vi "Main.vi"() -> ()   [LabVIEW 2018, in "Application.lvlib"]
doc: "This VI is the main application VI in the Delacor QMH project template. This application VI is implemented as a simple state machine, which communicates with two different Delacor QMH modules.\n_____\nBased on DQMH Project Template 6.0.0.91."
uses:
  Application.lvlib
  Application Data--cluster.ctl
  State--enum.ctl
  CE14 eMIC module/CE14 eMIC module.lvlib
  Switches Module/Switches Module.lvlib
panel:
  in  "Array":bool[](array[boolean])
  in  "MB01":bool
  in  "CloseCOM":bool
  in  "OpenCOM":bool
  out "version":string
  in  "Hide Switches Module Module":bool
  in  "Show Switches Module Module":bool
  in  "Hide CE14 eMIC module Module":bool
  in  "Show CE14 eMIC module Module":bool
  in  "Stop CE14 eMIC module Module":bool
  in  "Stop Switches Module Module":bool
  in  "Start Switches Module Module":bool
  out "Active CE14 eMIC module Modules":string[](array[string])
  in  "Start New Instance CE14 eMIC module Module":bool
  in  "Select CE14 eMIC module Module Instance":i32(ring)=-1 items=["All"=-1]
  in  "Switches Module Module: Do Something Else":dbl caption="Do Something Else"
  in  "Switches Module Module: Do Something":bool
  out "Switches Module Running?":bool
  out "Status":string
  in  "CE14 eMIC module Module: Do Something Else":dbl caption="Do Something Else to Selected Module"
  in  "CE14 eMIC module Module: Do Something":bool caption="Do Something to Selected Module"
  # "This top-level application allows you to launch and control a singleton module, and multiple instances of a cloneable module."
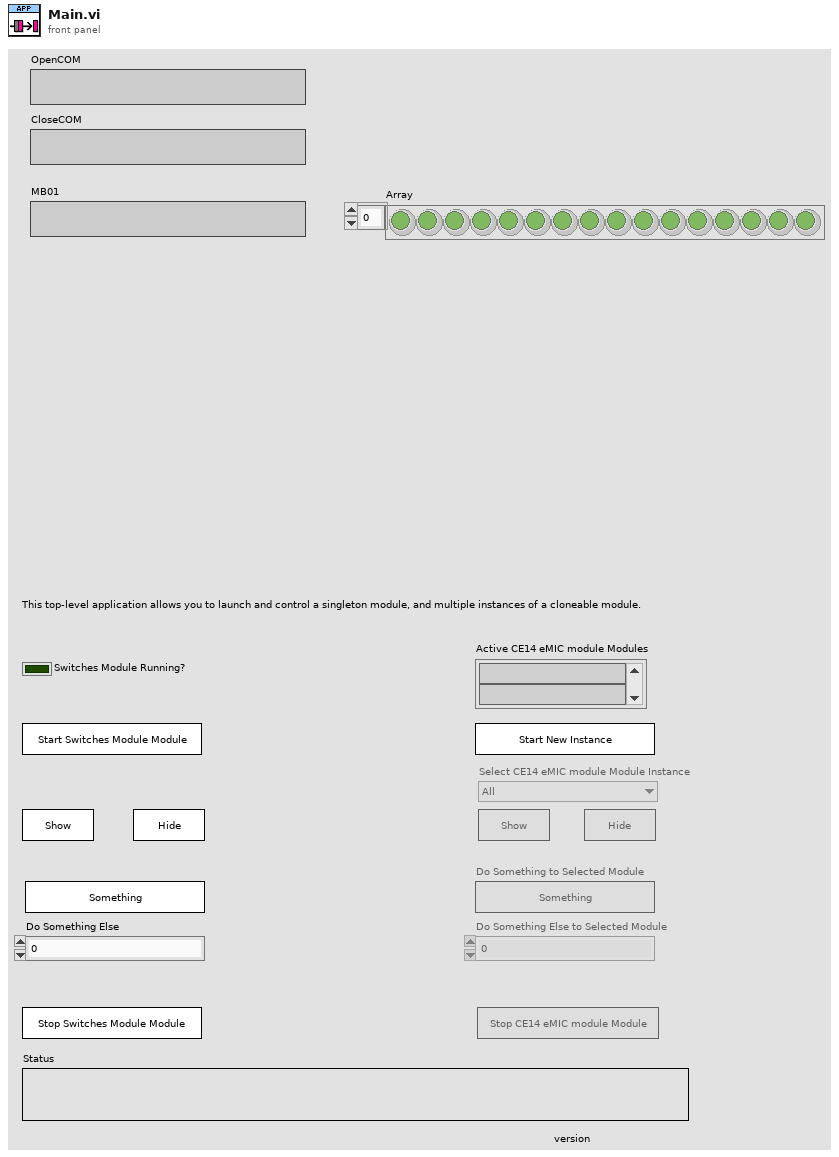
[diagram p1: front panel]
types:
  T1 = typedef "Application.lvlib/State--enum.ctl" = enum16{"Initialize", "Initialize Panel", "UI Interlocks", "Update Status", "Wait for Event", "Exit"}
  T2 = typedef "Application.lvlib/Application Data--cluster.ctl" = cluster{"Status":string, "Singleton Controls":refnum<vi>[], "Cloneable Controls":refnum<vi>[], "Module Ring Value":i32}
  T3 = typedef "CE14 eMIC module.lvlib/Broadcast Events--cluster.ctl" = cluster{"Module Did Init":refnum<user-event>, "Status Updated":refnum<user-event>, "Error Reported":refnum<user-event>, "Did Something":refnum<user-event>, "Module Did Stop":refnum<user-event>, "Update Module Execution Status":refnum<user-event>}
  T4 = typedef "Switches Module.lvlib/Broadcast Events--cluster.ctl" = cluster{"Module Did Init":refnum<user-event>, "Status Updated":refnum<user-event>, "Error Reported":refnum<user-event>, "Did Something":refnum<user-event>, "Module Did Stop":refnum<user-event>, "Update Module Execution Status":refnum<user-event>}
  T5 = enum8{"Enabled", "Disabled", "Disabled and Grayed Out"}
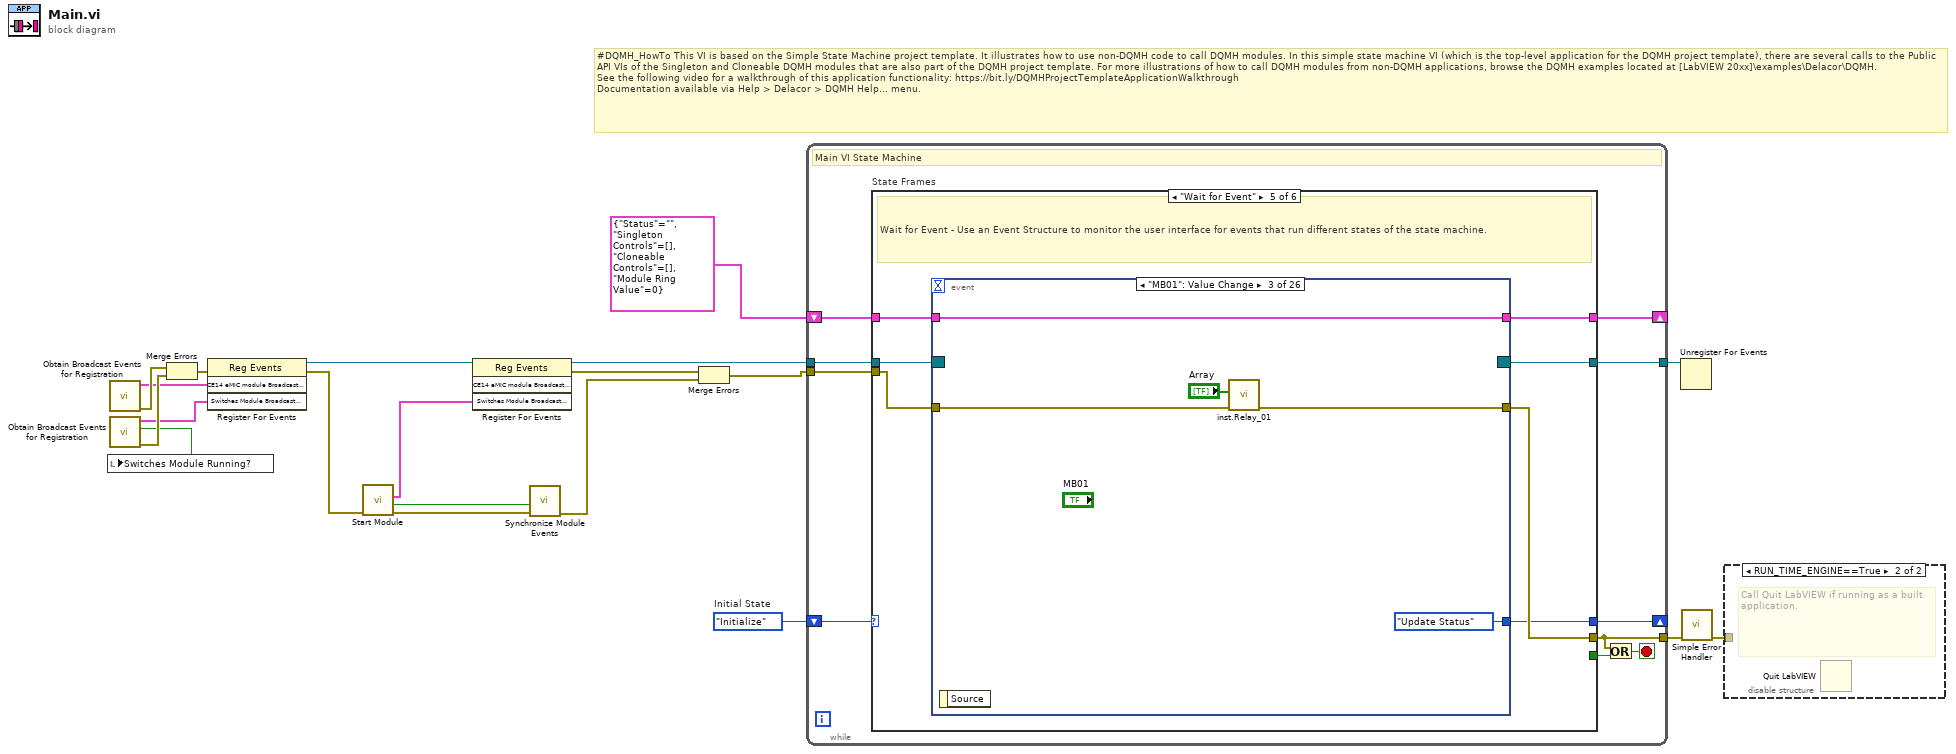
[diagram p0: block diagram]
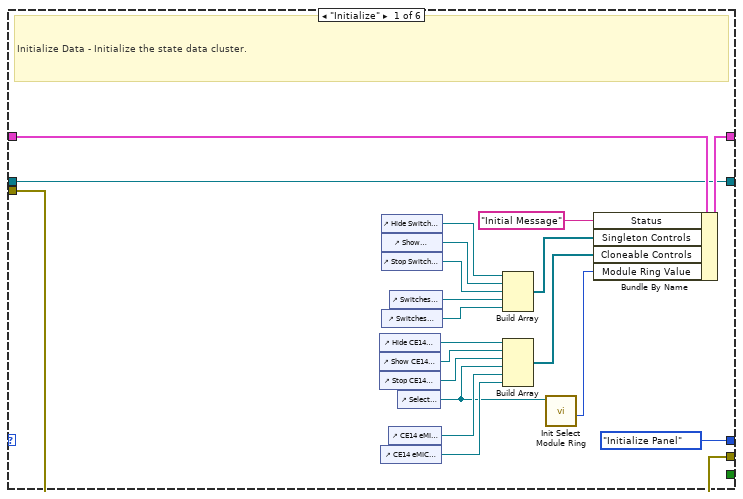
[diagram p2: hidden frame]
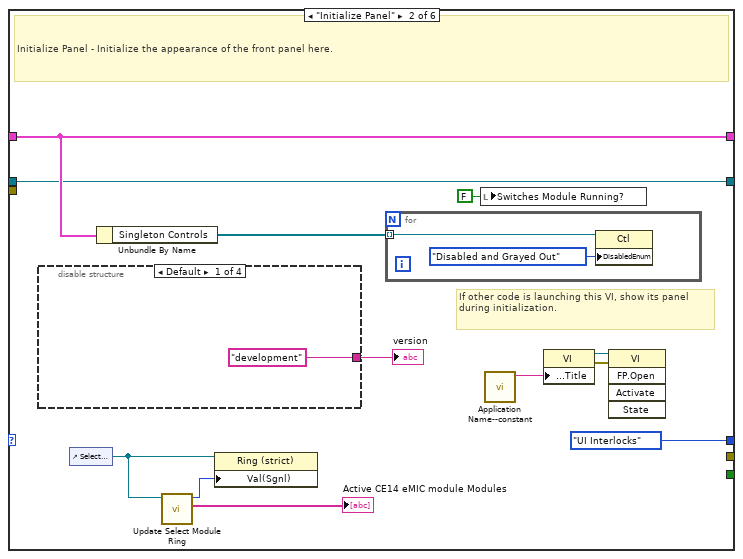
[diagram p3: hidden frame]
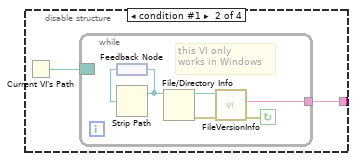
[diagram p4: hidden frame]
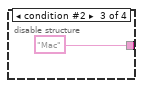
[diagram p5: hidden frame]
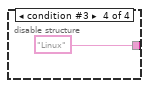
[diagram p6: hidden frame]
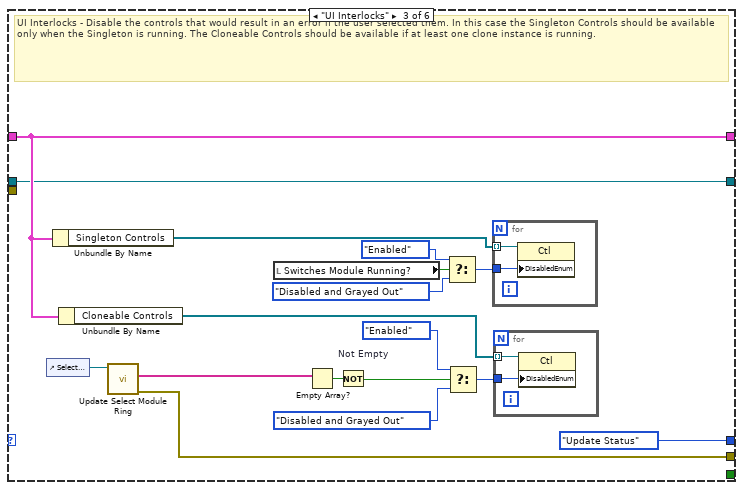
[diagram p7: hidden frame]
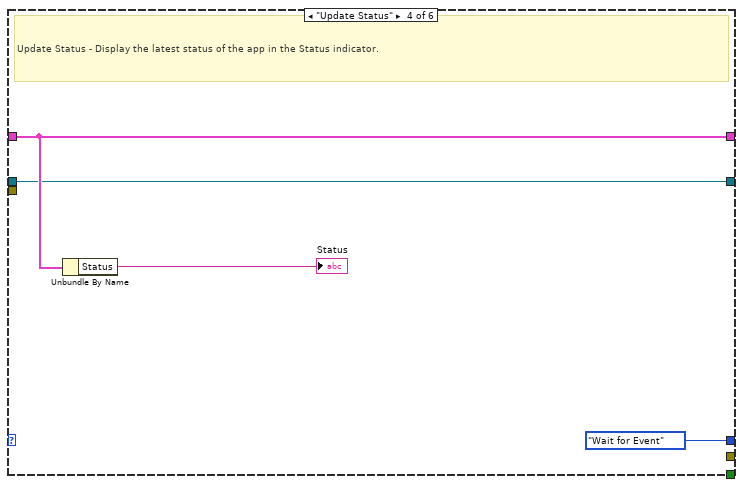
[diagram p8: hidden frame]
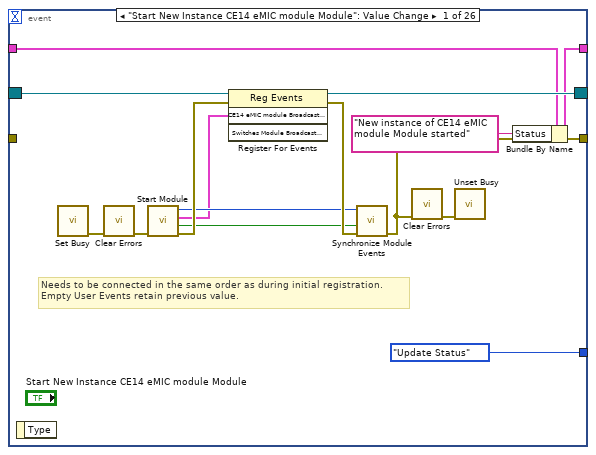
[diagram p9: hidden frame]
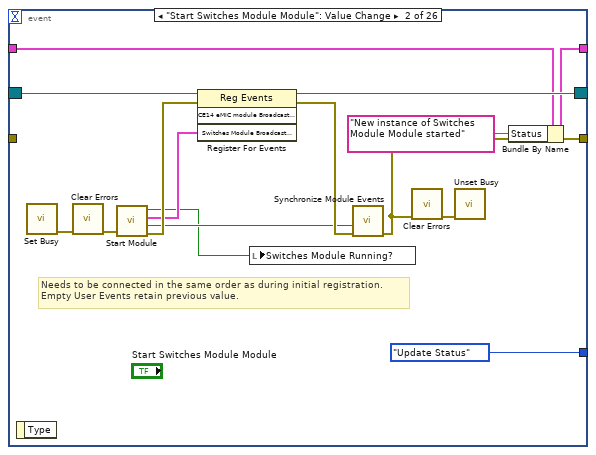
[diagram p10: hidden frame]
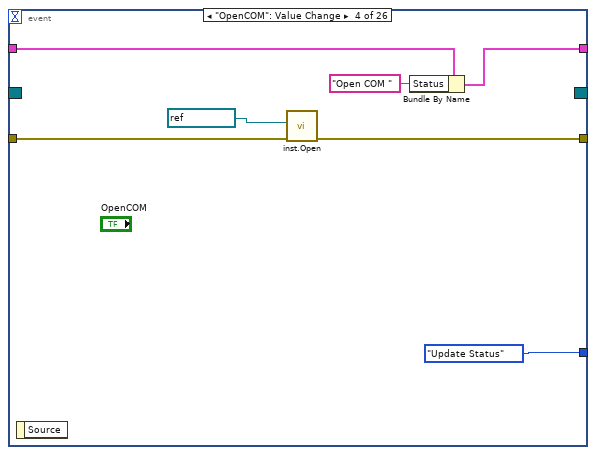
[diagram p11: hidden frame]
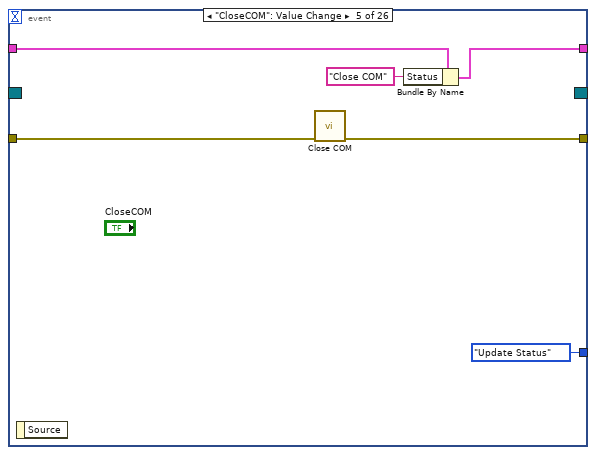
[diagram p12: hidden frame]
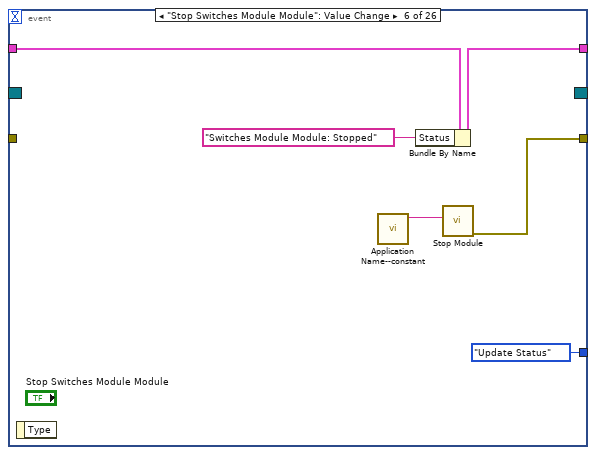
[diagram p13: hidden frame]
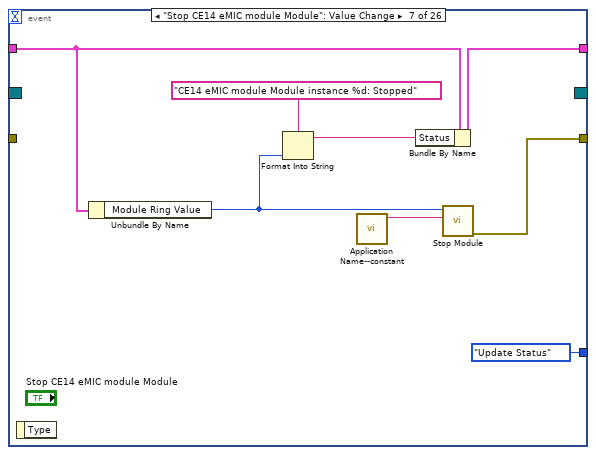
[diagram p14: hidden frame]
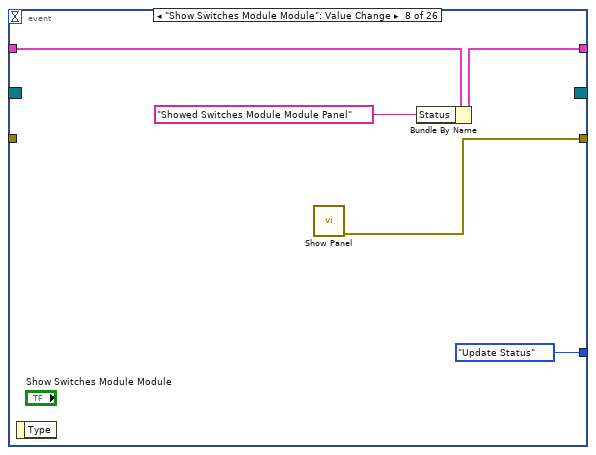
[diagram p15: hidden frame]
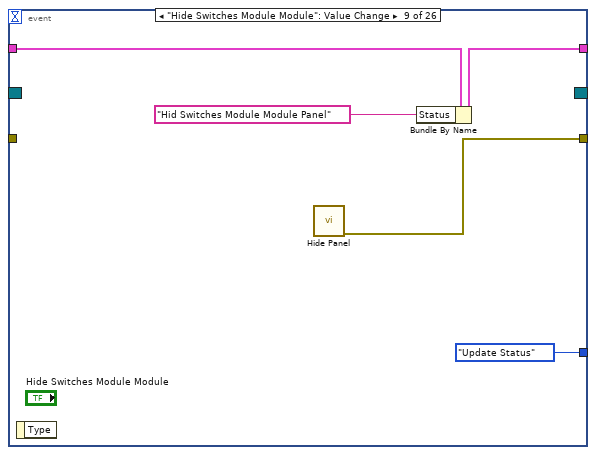
[diagram p16: hidden frame]
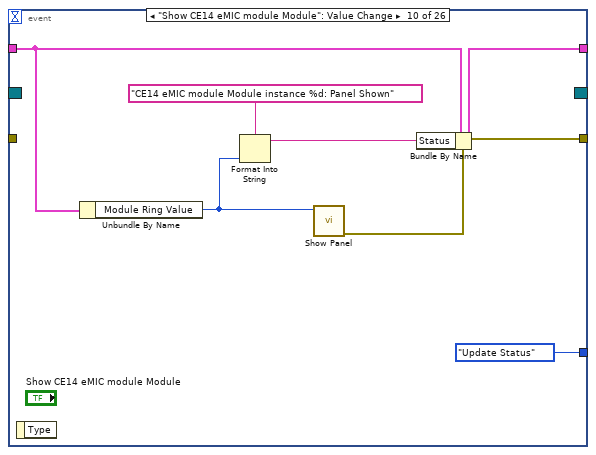
[diagram p17: hidden frame]
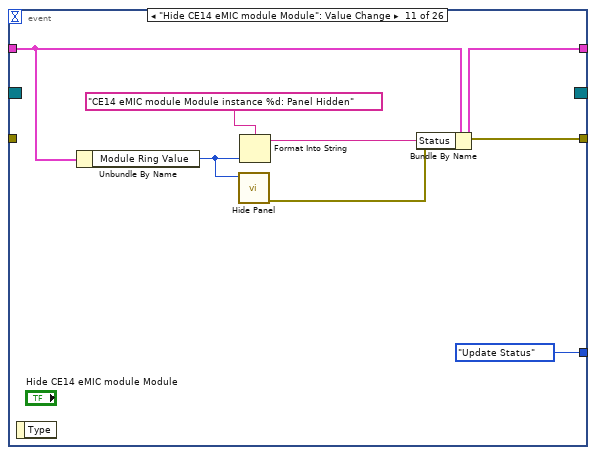
[diagram p18: hidden frame]
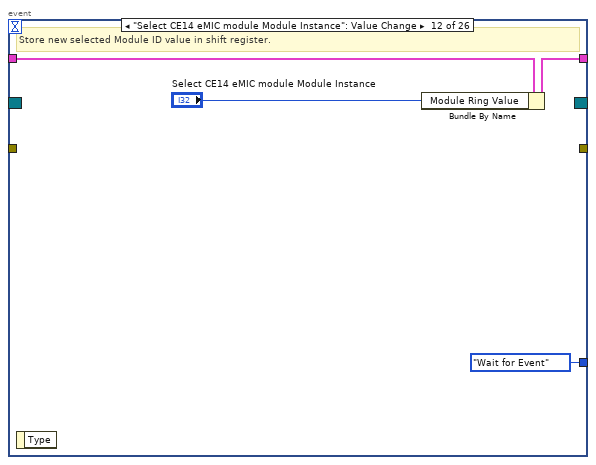
[diagram p19: hidden frame]
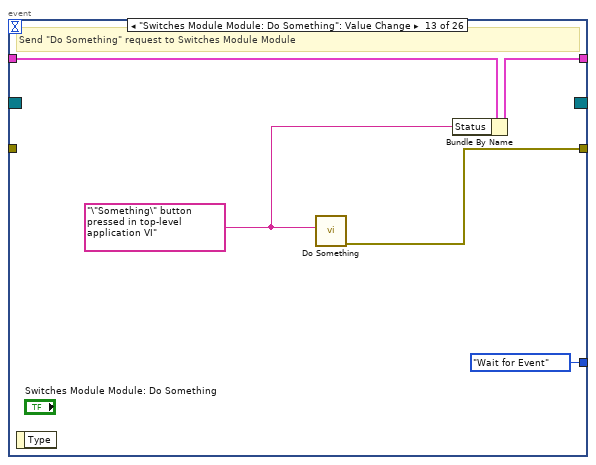
[diagram p20: hidden frame]
diagram:
  w12 = State--enum."Initialize"  # Initial State
  # "#DQMH_HowTo This VI is based on the Simple State Machine project template. It illustrates how to use non-DQMH code to call DQMH modules. In this simple state machine VI (which is the top-level application for the DQMH project template), there are several calls to the Public API VIs of the Singleton and Cloneable DQMH modules that are also part of the DQMH project template. For more illustrations of how to call DQMH modules from non-DQMH applications, browse the DQMH examples located at [LabVIEW 20xx]\\examples\\Delacor\\DQMH.\nSee the following video for a walkthrough of this application functionality: https://bit.ly/DQMHProjectTemplateApplicationWalkthrough\nDocumentation available via Help > Delacor > DQMH Help... menu."
  n1 = call "Obtain Broadcast Events for Registration.vi"() -> ("error out"=w17:errorcluster, "CE14 eMIC module Broadcast Events"=w14:T3)  [unwired: 9 in, 1 out]
  n2 = call "Obtain Broadcast Events for Registration.vi"() -> ("error out"=w16:errorcluster, "Already running?"=w10:bool, "Switches Module Broadcast Events"=w13:T4)  [unwired: 9 in]
  n3 = local write "Switches Module Running?"(w10) -> ()
  n4 = Merge Errors(w17, w16) -> (w18:errorcluster)
  n5 = register-events(error in=w18, w14, w13) -> (reference out=w7:refnum<event-registration>, error out=w8:errorcluster)  [unwired: 1 in]
  n6 = call "Start Module.vi"("error in (no error)"=w8) -> ("error out"=w9:errorcluster, "Wait for Event Sync?"=w6:bool, "Switches Module Broadcast Events"=w5:T4)  [unwired: 7 in, 1 out]
  n7 = register-events(reference=w7, w5) -> (reference out=w4:refnum<event-registration>, error out=w3:errorcluster)  [unwired: 2 in]
  n8 = call "Synchronize Module Events.vi"("error in"=w9, "Wait for Event Sync?"=w6) -> ("error out"=w2:errorcluster)  [unwired: 9 in]
  n9 = Merge Errors(w3, w2) -> (w1:errorcluster)
  n10 = while {
    shift-right: [w27] -> _
    shift-left: T2 {"Status"="", "Singleton Controls"=[], "Cloneable Controls"=[], "Module Ring Value"=0} ("Data Cluster") -> [w28]
    tunnel: [w30] -> w20
    shift-right: [w23] -> _
    shift-left: w12 -> [w25]
    tunnel: w1 -> [w29]
    tunnel: w4 -> [w22]
    tunnel: [w21] -> w11
    stop <- w24 stop-if-true
    # "Main VI State Machine"
    n11 = case "State Frames" shown="\"Wait for Event\"" w25 {
      tunnel: [w50 _ w92 _ w107 w296] -> w30
      tunnel: w28 -> [w49 w59 w80 w100 w104 w293]
      tunnel: [w48 w59 w80 w100 w103 w293] -> w27
      tunnel: [_ _ _ _ _ w292] -> w26
      tunnel: [State--enum."Initialize Panel" ("State") State--enum."UI Interlocks" ("State") State--enum."Update Status" ("State") State--enum."Wait for Event" ("State") w102 State--enum."Exit" ("State")] -> w23
      tunnel: w22 -> [w31 w56 w76 w97 w106 w290]
      tunnel: [w31 w56 w76 w97 w105 w290] -> w21
      tunnel: w29 -> [w50 _ _ _ w101 _]
      frame "Initialize" {
        # "Initialize Data - Initialize the state data cluster."
        n12 = control-ref of="Hide CE14 eMIC module Module"() -> (w40:refnum<vi>)
        n13 = control-ref of="Show CE14 eMIC module Module"() -> (w39:refnum<vi>)
        n14 = control-ref of="Stop CE14 eMIC module Module"() -> (w38:refnum<vi>)
        n15 = control-ref of="CE14 eMIC module Module: Do Something"() -> (w35:refnum<vi>)
        n16 = control-ref of="Hide Switches Module Module"() -> (w46:refnum<vi>)
        n17 = control-ref of="Show Switches Module Module"() -> (w45:refnum<vi>)
        n18 = control-ref of="Stop Switches Module Module"() -> (w44:refnum<vi>)
        n19 = control-ref of="Switches Module Module: Do Something"() -> (w42:refnum<vi>)
        n20 = control-ref of="CE14 eMIC module Module: Do Something Else"() -> (w36:refnum<vi>)
        n21 = control-ref of="Switches Module Module: Do Something Else"() -> (w43:refnum<vi>)
        n22 = control-ref of="Select CE14 eMIC module Module Instance"() -> (w33:refnum<vi>)
        n23 = Build Array(w46, w45, w44, w43, w42) -> (w41:refnum<vi>[])
        n24 = Build Array(w40, w39, w38, w33, w36, w35) -> (w37:refnum<vi>[])
        n25 = call "Init Select Module Ring.vi"("Select Module Ring Ref"=w33) -> ("Module Ring Value"=w32:i32)  [unwired: 8 in, 2 out]
        n26 = Bundle By Name(cluster=w49, "Status"="Initial Message" ("Initial Message"), "Singleton Controls"=w41, "Cloneable Controls"=w37, "Module Ring Value"=w32) -> (w48:T2)
      }
      frame "Initialize Panel" {
        # "If other code is launching this VI, show its panel during initialization."
        # "Initialize Panel - Initialize the appearance of the front panel here."
        n27 = disable-structure "Conditional Disable Structure" shown="Default" {
          disable-tunnel: ["development" w64 "Mac" "Linux"] -> w53
          frame condition #0 (active) {
          }
          frame condition #1 {
            n28 = Current VI's Path() -> (path=w65:path)
            n29 = while {
              border: w65 -> [_]
              tunnel: [w66] -> w64
              stop <- w70 continue-if-true
              # "this VI only \nworks in Windows"
              n30 = feedback #1() -> (w69:path)
              n31 = Strip Path(path=w69) -> (stripped path=w68:path)  [unwired: 1 out]
              n32 = feedback-in #1(w68) -> ()
              n33 = File/Directory Info(path=w68) -> (path out=w67:path, error out=w71:errorcluster)  [unwired: 1 in, 5 out]
              n34 = call <vilib>:"FileVersionInfo.vi"("error in (no error)"=w71, "Application Path in"=w67) -> ("error out"=w70:errorcluster, "File Version Info"=w66:string)  [unwired: 6 in, 2 out]
            }
          }
          frame condition #2 {
          }
          frame condition #3 {
          }
        }
        "version" <- w53
        n35 = control-ref of="Select CE14 eMIC module Module Instance"() -> (w55:refnum<vi>)
        n36 = Unbundle By Name(w59) -> ("Singleton Controls"=w58:refnum<vi>[])
        n37 = call "Update Select Module Ring.vi"("Select Module Ring Ref"=w55) -> ("Active Modules (Array)"=→"Active CE14 eMIC module Modules":string[], "New Module Ring Value"=w54:i32)  [unwired: 8 in, 1 out]
        n38 = property on="Property Node" class="Ring (strict)"(reference=w55, "Val(Sgnl)"=w54) -> ()  [unwired: 1 in, 2 out]
        n39 = for {
          tunnel: w58 -> [w75] mode=indexing
          n40 = property on="Property Node" class="Ctl"(reference=w75, "DisabledEnum"=T5."Disabled and Grayed Out" ("Disabled")) -> ()  [unwired: 1 in, 2 out]
        }
        n41 = local write "Switches Module Running?"(FALSE ("My Singleton Module Init?")) -> ()
        n42 = call "Application Name--constant.vi"() -> ("Application Name"=w52:string)  [unwired: 11 in]
        n43 = property on="Property Node" class="VI"("Front Panel.Title"=w52) -> (reference out=w51:refnum<vi>, error out=w62:errorcluster)  [unwired: 2 in]
        n44 = invoke class="VI" method="FP.Open"(reference=w51, error in=w62) -> ()  [unwired: 3 in, 5 out]
      }
      frame "UI Interlocks" {
        # "UI Interlocks - Disable the controls that would result in an error if the user selected them. In this case the Singleton Controls should be available only when the Singleton is running. The Cloneable Controls should be available if at least one clone instance is running."
        n45 = control-ref of="Select CE14 eMIC module Module Instance"() -> (w91:refnum<vi>)
        n46 = Unbundle By Name(w80) -> ("Singleton Controls"=w85:refnum<vi>[])
        n47 = Unbundle By Name(w80) -> ("Cloneable Controls"=w79:refnum<vi>[])
        n48 = call "Update Select Module Ring.vi"("Select Module Ring Ref"=w91) -> ("error out"=w92:errorcluster, "Active Modules (Array)"=w90:string[])  [unwired: 8 in, 1 out]
        n49 = local read "Switches Module Running?"() -> (w84:bool)
        n50 = Empty Array?(array=w90) -> (empty?=w89:bool)
        n51 = Not "Not Empty"(x=w89) -> (.not. x?=w78:bool)
        n52 = Select(t=T5."Enabled" ("Disabled"), s=w84, f=T5."Disabled and Grayed Out" ("Disabled")) -> (s? t:f=w86:T5)
        n53 = Select(t=T5."Enabled" ("Disabled"), s=w78, f=T5."Disabled and Grayed Out" ("Disabled")) -> (s? t:f=w83:T5)
        n54 = for {
          tunnel: w85 -> [w96] mode=indexing
          tunnel: w86 -> [w95]
          n55 = property on="Property Node" class="Ctl"(reference=w96, "DisabledEnum"=w95) -> ()  [unwired: 1 in, 2 out]
        }
        n56 = for {
          tunnel: w79 -> [w94] mode=indexing
          tunnel: w83 -> [w93]
          n57 = property on="Property Node" class="Ctl"(reference=w94, "DisabledEnum"=w93) -> ()  [unwired: 1 in, 2 out]
        }
      }
      frame "Update Status" {
        # "Update Status - Display the latest status of the app in the Status indicator."
        n58 = Unbundle By Name(w100) -> ("Status"=→"Status":string)
      }
      frame "Wait for Event" {
        # "Wait for Event - Use an Event Structure to monitor the user interface for events that run different states of the state machine."
        n59 = event shown="[2] \"MB01\": Value Change" {
          selector: w106 -> [w114 w130 _ _ _ _ _ _ _ _ _ _ _ _ _ _ _ _ _ _ _ _ _ _ _ _]
          dyn-events: [w113 w129 _ _ _ _ _ _ _ _ _ _ _ _ _ _ _ _ _ _ _ _ _ _ _ _] -> w105
          timeout: _ -> [_ _ _ _ _ _ _ _ _ _ _ _ _ _ _ _ _ _ _ _ _ _ _ _ _ _]
          tunnel: [w122 w137 w139 w148 w154 w161 w169 w174 w179 w186 w193 _ w202 w208 w214 w221 w229 w234 w238 _ _ _ _ w276 _ _] -> w107
          tunnel: [w109 w126 w142 w144 w152 w157 w166 w172 w177 w185 w192 w195 w200 w207 w212 w220 w223 w231 w237 w240 w245 w255 w265 w269 w280 w285] -> w103
          tunnel: w104 -> [w110 w127 w142 w143 w151 w158 w165 w173 w178 w183 w190 w196 w201 w204 w213 w218 w223 w231 w237 w241 w246 w256 w266 w272 w281 w285]
          tunnel: [State--enum."Update Status" ("State") State--enum."Update Status" ("State") State--enum."Update Status" ("State") State--enum."Update Status" ("State") State--enum."Update Status" ("State") State--enum."Update Status" ("State") State--enum."Update Status" ("State") State--enum."Update Status" ("State") State--enum."Update Status" ("State") State--enum."Update Status" ("State") State--enum."Update Status" ("State") State--enum."Wait for Event" ("State") State--enum."Wait for Event" ("State") State--enum."Wait for Event" ("State") State--enum."Update Status" ("State") State--enum."Update Status" ("State") State--enum."UI Interlocks" ("State") State--enum."UI Interlocks" ("State") State--enum."UI Interlocks" ("State") State--enum."Update Status" ("State") State--enum."Update Status" ("State") State--enum."Update Status" ("State") State--enum."Update Status" ("State") State--enum."UI Interlocks" ("State") State--enum."UI Interlocks" ("State") State--enum."Exit" ("State")] -> w102
          tunnel: w101 -> [_ _ w140 w149 w155 _ _ _ _ _ _ _ _ _ _ _ _ _ _ _ _ _ _ _ _ _]
          event "Start New Instance CE14 eMIC module Module": Value Change {
            # "Needs to be connected in the same order as during initial registration.\nEmpty User Events retain previous value."
            n60 = event-data() -> ()  [unwired: 1 in, 1 out]
            n61 = call <vilib>:"Set Busy.vi"() -> ("error out"=w118:errorcluster)  [unwired: 10 in, 1 out]
            n62 = call <vilib>:"Clear Errors.vi"("error in (no error)"=w118) -> ("error out"=w119:errorcluster)  [unwired: 5 in, 1 out]
            n63 = call "Start Module.vi"("error in"=w119) -> ("error out"=w121:errorcluster, "Wait for Event Sync?"=w116:bool, "CE14 eMIC module Broadcast Events"=w112:T3, "Module ID"=w115:i32)  [unwired: 7 in]
            n64 = register-events(reference=w114, error in=w121, w112) -> (reference out=w113:refnum<event-registration>, error out=w120:errorcluster)  [unwired: 1 in]
            n65 = call "Synchronize Module Events.vi"("error in"=w120, "Wait for Event Sync?"=w116, "Module ID in"=w115) -> ("error out"=w122:errorcluster)  [unwired: 7 in, 1 out]
            n66 = call <vilib>:"Clear Errors.vi"("error in (no error)"=w122) -> ("error out"=w117:errorcluster)  [unwired: 5 in, 1 out]
            n67 = call <vilib>:"Unset Busy.vi"("error in (no error)"=w117) -> ()  [unwired: 10 in, 1 out]
            n68 = Bundle By Name(cluster=w110, "Status"="New instance of CE14 eMIC module Module started") -> (w109:T2)
          }
          event "Start Switches Module Module": Value Change {
            # "Needs to be connected in the same order as during initial registration.\nEmpty User Events retain previous value."
            n69 = event-data() -> ()  [unwired: 1 in, 1 out]
            n70 = call <vilib>:"Set Busy.vi"() -> ("error out"=w133:errorcluster)  [unwired: 10 in, 1 out]
            n71 = call <vilib>:"Clear Errors.vi"("error in (no error)"=w133) -> ("error out"=w134:errorcluster)  [unwired: 5 in, 1 out]
            n72 = call "Start Module.vi"("error in (no error)"=w134) -> ("error out"=w136:errorcluster, "Wait for Event Sync?"=w131:bool, "Switches Module Broadcast Events"=w124:T4, "Module Was Already Running?"=w123:bool)  [unwired: 7 in]
            n73 = register-events(reference=w130, error in=w136, w124) -> (reference out=w129:refnum<event-registration>, error out=w135:errorcluster)  [unwired: 1 in]
            n74 = local write "Switches Module Running?"(w123) -> ()
            n75 = call "Synchronize Module Events.vi"("error in"=w135, "Wait for Event Sync?"=w131) -> ("error out"=w137:errorcluster)  [unwired: 9 in]
            n76 = call <vilib>:"Clear Errors.vi"("error in (no error)"=w137) -> ("error out"=w132:errorcluster)  [unwired: 5 in, 1 out]
            n77 = call <vilib>:"Unset Busy.vi"("error in (no error)"=w132) -> ()  [unwired: 10 in, 1 out]
            n78 = Bundle By Name(cluster=w127, "Status"="New instance of Switches Module Module started") -> (w126:T2)
          }
          event "MB01": Value Change {
            n79 = event-data() -> ()  [unwired: 1 in, 1 out]
            n80 = call "inst.Relay_01.vi"("error in"=w140, "Array"="Array") -> ("error out"=w139:errorcluster)  [unwired: 9 in]
          }
          event "OpenCOM": Value Change {
            n81 = event-data() -> ()  [unwired: 1 in, 1 out]
            n82 = call "inst.Open.vi"("error in"=w149, "VISA resource name"=refnum<visa-resource-name> "COM11") -> ("error out"=w148:errorcluster)  [unwired: 9 in]
            n83 = Bundle By Name(cluster=w143, "Status"="Open COM ") -> (w144:T2)
          }
          event "CloseCOM": Value Change {
            n84 = event-data() -> ()  [unwired: 1 in, 1 out]
            n85 = call "Close COM.vi"("error in"=w155) -> ("error out"=w154:errorcluster)  [unwired: 10 in]
            n86 = Bundle By Name(cluster=w151, "Status"="Close COM") -> (w152:T2)
          }
          event "Stop Switches Module Module": Value Change {
            n87 = event-data() -> ()  [unwired: 1 in, 1 out]
            n88 = call "Application Name--constant.vi"() -> ("Application Name"=w159:string)  [unwired: 11 in]
            n89 = Bundle By Name(cluster=w158, "Status"="Switches Module Module: Stopped" ("Message")) -> (w157:T2)
            n90 = call "Stop Module.vi"("Origin"=w159) -> ("error out"=w161:errorcluster)  [unwired: 10 in]
          }
          event "Stop CE14 eMIC module Module": Value Change {
            n91 = event-data() -> ()  [unwired: 1 in, 1 out]
            n92 = Unbundle By Name(w165) -> ("Module Ring Value"=w162:i32)
            n93 = Format Into String(format string="CE14 eMIC module Module instance %d: Stopped" ("Message"), w162) -> (resulting string=w163:string)  [unwired: 2 in, 1 out]
            n94 = call "Application Name--constant.vi"() -> ("Application Name"=w167:string)  [unwired: 11 in]
            n95 = Bundle By Name(cluster=w165, "Status"=w163) -> (w166:T2)
            n96 = call "Stop Module.vi"("Origin"=w167, "Module ID"=w162) -> ("error out"=w169:errorcluster)  [unwired: 9 in]
          }
          event "Show Switches Module Module": Value Change {
            n97 = event-data() -> ()  [unwired: 1 in, 1 out]
            n98 = call "Show Panel.vi"() -> ("error out"=w174:errorcluster)  [unwired: 11 in]
            n99 = Bundle By Name(cluster=w173, "Status"="Showed Switches Module Module Panel" ("Message")) -> (w172:T2)
          }
          event "Hide Switches Module Module": Value Change {
            n100 = event-data() -> ()  [unwired: 1 in, 1 out]
            n101 = call "Hide Panel.vi"() -> ("error out"=w179:errorcluster)  [unwired: 11 in]
            n102 = Bundle By Name(cluster=w178, "Status"="Hid Switches Module Module Panel" ("Message")) -> (w177:T2)
          }
          event "Show CE14 eMIC module Module": Value Change {
            n103 = event-data() -> ()  [unwired: 1 in, 1 out]
            n104 = Unbundle By Name(w183) -> ("Module Ring Value"=w181:i32)
            n105 = Format Into String(format string="CE14 eMIC module Module instance %d: Panel Shown" ("Message"), w181) -> (resulting string=w180:string)  [unwired: 2 in, 1 out]
            n106 = call "Show Panel.vi"("Module ID"=w181) -> ("error out"=w186:errorcluster)  [unwired: 10 in]
            n107 = Bundle By Name(cluster=w183, "Status"=w180) -> (w185:T2)
          }
          event "Hide CE14 eMIC module Module": Value Change {
            n108 = event-data() -> ()  [unwired: 1 in, 1 out]
            n109 = Unbundle By Name(w190) -> ("Module Ring Value"=w188:i32)
            n110 = call "Hide Panel.vi"("Module ID"=w188) -> ("error out"=w193:errorcluster)  [unwired: 10 in]
            n111 = Format Into String(format string="CE14 eMIC module Module instance %d: Panel Hidden" ("Message"), w188) -> (resulting string=w187:string)  [unwired: 2 in, 1 out]
            n112 = Bundle By Name(cluster=w190, "Status"=w187) -> (w192:T2)
          }
          event "Select CE14 eMIC module Module Instance": Value Change {
            # "Store new selected Module ID value in shift register."
            n113 = event-data() -> ()  [unwired: 1 in, 1 out]
            n114 = Bundle By Name(cluster=w196, "Module Ring Value"="Select CE14 eMIC module Module Instance") -> (w195:T2)
          }
          event "Switches Module Module: Do Something": Value Change {
            w199 = "\"Something\" button pressed in top-level application VI" ("\"Do Something Else\" button pressed")
            # "Send \"Do Something\" request to Switches Module Module"
            n115 = event-data() -> ()  [unwired: 1 in, 1 out]
            n116 = call "Do Something.vi"("Do Something Message"=w199) -> ("error out"=w202:errorcluster)  [unwired: 10 in]
            n117 = Bundle By Name(cluster=w201, "Status"=w199) -> (w200:T2)
          }
          event "CE14 eMIC module Module: Do Something": Value Change {
            w206 = "\"Something\" button pressed in top-level application VI" ("\"Do Something Else\" button pressed")
            # "Send \"Do Something\" request to CE14 eMIC module Module"
            n118 = event-data() -> ()  [unwired: 1 in, 1 out]
            n119 = Unbundle By Name(w204) -> ("Module Ring Value"=w203:i32)
            n120 = call "Do Something.vi"("Do Something Message"=w206, "Module ID"=w203) -> ("error out"=w208:errorcluster)  [unwired: 9 in]
            n121 = Bundle By Name(cluster=w204, "Status"=w206) -> (w207:T2)
          }
          event "Switches Module Module: Do Something Else": Value Change {
            w209 = "\"Do Something Else\" numeric value changed in top-level application VI. New value: " ("\"Do Something Else\" button pressed")
            # "Send \"Do Something Else\" request to Switches Module Module"
            n122 = event-data() -> ()  [unwired: 1 in, 1 out]
            n123 = call "Do Something Else.vi"("X"="Switches Module Module: Do Something Else", "Do Something Else Message"=w209) -> ("error out"=w214:errorcluster)  [unwired: 9 in]
            n124 = Bundle By Name(cluster=w213, "Status"=w209) -> (w212:T2)
          }
          event "CE14 eMIC module Module: Do Something Else": Value Change {
            w215 = "\"Do Something Else\" numeric value changed in top-level application VI. New value: " ("\"Do Something Else\" button pressed")
            # "Send \"Do Something Else\" request to CE14 eMIC module Module"
            n125 = event-data() -> ()  [unwired: 1 in, 1 out]
            n126 = Unbundle By Name(w218) -> ("Module Ring Value"=w217:i32)
            n127 = call "Do Something Else.vi"("X"="CE14 eMIC module Module: Do Something Else", "Do Something else Message"=w215, "Module ID"=w217) -> ("error out"=w221:errorcluster)  [unwired: 8 in]
            n128 = Bundle By Name(cluster=w218, "Status"=w215) -> (w220:T2)
          }
          event User Event {
            # "A new instance of CE14 eMIC module Module has broadcast that is has been initialized"
            n129 = event-data() -> ("Info"=w227:string, "Module ID"=w222:i32)  [unwired: 1 in]
            n130 = control-ref of="Select CE14 eMIC module Module Instance"() -> (w226:refnum<vi>)
            n131 = local write "Status"(w227) -> ()
            n132 = call "Update Select Module Ring.vi"("Select Module Ring Ref"=w226) -> ("error out"=w228:errorcluster, "Active Modules (Array)"=w225:string[])  [unwired: 8 in, 1 out]
            n133 = local write "Active CE14 eMIC module Modules"(w225) -> ()
            n134 = call "Show Panel.vi"("error in (no error)"=w228, "Module ID"=w222) -> ("error out"=w229:errorcluster)  [unwired: 9 in]
          }
          event User Event {
            # "Switches Module Module has broadcast that it has been initialized"
            n135 = event-data() -> ("Init?"=→"Switches Module Running?":bool, "Info"=w233:string)  [unwired: 1 in]
            n136 = local write "Status"(w233) -> ()
            n137 = call "Show Panel.vi"() -> ("error out"=w234:errorcluster)  [unwired: 11 in]
          }
          event User Event {
            # "Switches Module Module has broadcast its execution status"
            n138 = event-data() -> ("Running?"=w235:bool)  [unwired: 1 in]
            n139 = local write "Switches Module Running?"(w235) -> ()
            n140 = case shown="True" w235 {
              tunnel: [_ w239] -> w238
              frame False {
              }
              frame True {
                n141 = call "Show Panel.vi"() -> ("error out"=w239:errorcluster)  [unwired: 11 in]
              }
            }
          }
          event User Event {
            # "An instance of CE14 eMIC module Module has broadcast its status"
            n142 = event-data() -> ("Status"=w243:string)  [unwired: 1 in]
            n143 = Bundle By Name(cluster=w241, "Status"=w243) -> (w240:T2)
          }
          event User Event {
            # "Switches Module Module has broadcast its status"
            n144 = event-data() -> ("Status"=w247:string)  [unwired: 1 in]
            n145 = Bundle By Name(cluster=w246, "Status"=w247) -> (w245:T2)
          }
          event User Event {
            # "CE14 eMIC module Module had an error"
            n146 = event-data() -> ("Module Name"=w249:string, "Additional Information"=w252:string, "Error"=w257:errorcluster)  [unwired: 1 in]
            n147 = Unbundle By Name(w257) -> ("code"=w248:i32, "source"=w251:string)
            n148 = Format Into String(format string="Error code %d  Module: %s Additional Information: %s\nSource: %s", w248, w249, w252, w251) -> (resulting string=w250:string)  [unwired: 2 in, 1 out]
            n149 = Bundle By Name(cluster=w256, "Status"=w250) -> (w255:T2)
          }
          event User Event {
            # "Switches Module Module had an error"
            n150 = event-data() -> ("Module Name"=w259:string, "Additional Information"=w263:string, "Error"=w267:errorcluster)  [unwired: 1 in]
            n151 = Unbundle By Name(w267) -> ("code"=w258:i32, "source"=w262:string)
            n152 = Format Into String(format string="Error code %d Module: %s  Additional Information: %s\nSource: %s", w258, w259, w263, w262) -> (resulting string=w260:string)  [unwired: 2 in, 1 out]
            n153 = Bundle By Name(cluster=w266, "Status"=w260) -> (w265:T2)
          }
          event User Event {
            n154 = event-data() -> ("Origin"=w271:string)  [unwired: 1 in]
            n155 = Bundle By Name(cluster=w272, "Status"=w271) -> (w270:T2)
            n156 = control-ref of="Select CE14 eMIC module Module Instance"() -> (w275:refnum<vi>)
            n157 = call "Update Select Module Ring.vi"("Select Module Ring Ref"=w275) -> ("error out"=w276:errorcluster, "Active Modules (Array)"=w274:string[], "New Module Ring Value"=w268:i32)  [unwired: 8 in]
            n158 = Bundle By Name(cluster=w270, "Module Ring Value"=w268) -> (w269:T2)
            n159 = local write "Active CE14 eMIC module Modules"(w274) -> ()
          }
          event User Event {
            n160 = event-data() -> ("Origin"=w278:string)  [unwired: 1 in]
            n161 = local write "Switches Module Running?"(FALSE ("My Singleton Module Init?")) -> ()
            n162 = Concatenate Strings(w278, " Did Stop.") -> (w277:string)
            n163 = Bundle By Name(cluster=w281, "Status"=w277) -> (w280:T2)
          }
          event Panel Close? {
            # "Go to the 'Exit' state if the user tries to close the panel."
            n164 = event-data() -> ()  [unwired: 1 in, 1 out]
            n165 = event-data ("Event Filter Node")("Discard?"=TRUE) -> ()  [unwired: 1 in, 1 out]
          }
        }
      }
      frame "Exit" {
        w287 = TRUE  # Wait for Module to stop?
        w292 = TRUE  # Stop the VI
        # "Stop all modules launched"
        # "Exit - Exit the application."
        n166 = call "Application Name--constant.vi"() -> ("Application Name"=w288:string)  [unwired: 11 in]
        n167 = call "Stop Module.vi"("Wait for Module to stop? (F)"=w287, "Origin"=w288, "Module ID"=-1) -> ("error out"=w294:errorcluster)  [unwired: 8 in]
        n168 = call "Stop Module.vi"("Wait for Module to Stop? (F)"=w287, "Origin"=w288) -> ("error out"=w295:errorcluster)  [unwired: 9 in]
        n169 = Merge Errors(w294, w295) -> (w296:errorcluster)
      }
    }
    n170 = Or(x=w30, y=w26) -> (x .or. y?=w24:bool)
  }
  n171 = Unregister For Events(event registration refnum=w11) -> ()  [unwired: 1 in, 1 out]
  n172 = call <vilib>:"Simple Error Handler.vi"("error in (no error)"=w20) -> ("error out"=w19:errorcluster)  [unwired: 4 in, 4 out]
  n173 = disable-structure "Conditional Disable Structure" shown="RUN_TIME_ENGINE==True" {
    disable-tunnel: w19 -> [_ _]
    frame condition #0 (active) {
    }
    frame condition #1 {
      # "Call Quit LabVIEW if running as a built application."
      n174 = Quit LabVIEW() -> ()  [unwired: 1 in]
    }
  }
